vi "StudentScope.vi"() -> ()   [LabVIEW 2015]
uses:
  <vilib>/DAQmx/read.llb/DAQmx Read (Analog 2D DBL NChan NSamp).vi
  <vilib>/DAQmx/create/channels.llb/DAQmx Create Channel (AI-Voltage-Basic).vi
  <vilib>/DAQmx/configure/timing.llb/DAQmx Timing (Sample Clock).vi
  <vilib>/DAQmx/miscellaneous.llb/DAQmx Fill In Error Info.vi
  <resource>/objmgr/daqmx.rc
panel:
  out "Hidden Power Spectrum":T1(graph)=[{"df"=0.0, "df"=2.0, "Power Spectrum (V^2 rms)"=array[5000 elements]}, {"df"=0.0, "df"=2.0, "Power Spectrum (V^2 rms)"=array[5000 elements]}]
  in  "CH B Center":bool
  in  "CH A Center":bool
  out "Hidden Scope":dbl[][](graph)
  out "Acq Rate (Hz)":dbl=20.0 caption="Acq Rate:" format="%#_2g"
  in  "Print":bool
  in  "Tab Control":enum32{"Scope", "Spectrum Analyzer"}(tab)
  out "dV":string="142.75 µs" caption="dV:"
  out "Scope graph":dbl[][](graph)=[[-0.0025862696478761516, 0.003794052366753585, -0.011518720468357783, 0.0025179879638276377, -0.01789904248298752, -0.010242656065431836, -0.016622978080061572, -0.008966591662505888, -0.0025862696478761516, 0.003794052366753585, 0.0025179879638276377, -0.0064144628566539935, -0.0013102052449502043, -0.011518720468357783, -0.003862334050802099, -0.008966591662505888, -0.003862334050802099, -0.0064144628566539935, -0.015346913677135626, 0.0025179879638276377, 0.0012419235609016904, -0.008966591662505888, -0.0064144628566539935, -0.008966591662505888, -0.003862334050802099, -0.003862334050802099, -0.016622978080061572, -0.010242656065431836, -0.0025862696478761516, -0.005138398453728046, -0.011518720468357783, 0.003794052366753585, -0.015346913677135626, -0.015346913677135626, 0.0025179879638276377, -0.0013102052449502043, -0.0064144628566539935, 0.003794052366753585, -0.016622978080061572, 0.0025179879638276377, -0.011518720468357783, -0.008966591662505888, -0.0025862696478761516, -0.008966591662505888, -0.0025862696478761516, -0.01279478487128373, -0.01279478487128373, -0.0013102052449502043, -0.011518720468357783, 0.003794052366753585, -0.0064144628566539935, -0.008966591662505888, -0.015346913677135626, -0.0025862696478761516, -0.003862334050802099, -0.0064144628566539935, -3.4140842024256955e-05, -0.005138398453728046, -0.011518720468357783, -0.005138398453728046, -0.007690527259579941, 0.007622245575531427, -0.007690527259579941, 0.007622245575531427, -0.0064144628566539935, -0.007690527259579941, -0.0025862696478761516, -0.0064144628566539935, -0.0064144628566539935, -0.0064144628566539935, -3.4140842024256955e-05, -0.007690527259579941, -0.01789904248298752, 0.0012419235609016904, -0.0064144628566539935, 0.003794052366753585, -0.011518720468357783, -0.003862334050802099, -0.015346913677135626, 0.003794052366753585, -0.011518720468357783, -0.007690527259579941, 0.005070116769679532, -0.0025862696478761516, -0.0013102052449502043, -0.008966591662505888, -0.003862334050802099, -0.0025862696478761516, -0.015346913677135626, -0.0064144628566539935, 0.0025179879638276377, 0.0012419235609016904, 0.003794052366753585, -0.01279478487128373, -0.016622978080061572, 0.0012419235609016904, -0.005138398453728046, 0.003794052366753585, -0.003862334050802099, -0.005138398453728046, -0.008966591662505888, -0.005138398453728046, 0.003794052366753585, 0.007622245575531427, -0.0064144628566539935, -0.008966591662505888, -0.0013102052449502043, -0.0064144628566539935, 0.014002567590161163, -0.010242656065431836, -0.010242656065431836, -0.008966591662505888, -0.016622978080061572, -0.0025862696478761516, -0.0025862696478761516, 0.005070116769679532, -0.016622978080061572, -0.0013102052449502043, -0.005138398453728046, -0.0013102052449502043, -0.0013102052449502043, 0.003794052366753585, 0.017830760798939006, -0.007690527259579941, -0.020451171288839415, -0.010242656065431836, -0.0013102052449502043, 0.005070116769679532, 0.014002567590161163, 0.007622245575531427, 0.00634618117260548, -0.011518720468357783, -0.0013102052449502043, -0.011518720468357783, -0.0025862696478761516, -0.0064144628566539935, -0.0025862696478761516, -0.0025862696478761516, 0.008898309978457374, 0.00634618117260548, -0.005138398453728046, 0.0025179879638276377, -0.008966591662505888, -0.007690527259579941, 0.005070116769679532, -0.0064144628566539935, 0.005070116769679532, -3.4140842024256955e-05, -0.005138398453728046, 0.0012419235609016904, -0.015346913677135626, 0.003794052366753585, -0.007690527259579941, 0.008898309978457374, 0.0025179879638276377, 0.0025179879638276377, -0.0013102052449502043, -3.4140842024256955e-05, 0.003794052366753585, 0.003794052366753585, -0.003862334050802099, 0.003794052366753585, -0.005138398453728046, -0.0064144628566539935, -0.008966591662505888, -0.0064144628566539935, -0.0013102052449502043, -0.007690527259579941, -3.4140842024256955e-05, -0.003862334050802099, 0.007622245575531427, 0.003794052366753585, 0.003794052366753585, -3.4140842024256955e-05, 0.003794052366753585, 0.003794052366753585, 0.008898309978457374, 0.012726503187235217, 0.0025179879638276377, -0.0025862696478761516, -0.0025862696478761516, -0.003862334050802099, -0.0013102052449502043, -0.0064144628566539935, -0.003862334050802099, 0.0025179879638276377, 0.008898309978457374, 0.005070116769679532, -0.0025862696478761516, 0.00634618117260548, 0.014002567590161163, -0.008966591662505888, 0.008898309978457374, 0.0025179879638276377, 0.014002567590161163, -0.0013102052449502043, 0.003794052366753585, -0.0025862696478761516, 0.01527863199308711, -0.005138398453728046], [-0.00392960120349739, 0.0037154429290138027, 0.0037154429290138027, -0.0013812531593269933, 0.006263790973184202, 0.0037154429290138027, 0.0037154429290138027, 0.006263790973184202, -0.00392960120349739, 0.0037154429290138027, 0.008812139017354599, -0.0013812531593269933, 0.0037154429290138027, 0.0037154429290138027, 0.0011670948848434039, 0.008812139017354599, 0.0037154429290138027, 0.0037154429290138027, 0.008812139017354599, -0.0013812531593269933, 0.0037154429290138027, 0.0037154429290138027, 0.0037154429290138027, 0.006263790973184202, -0.0013812531593269933, 0.0011670948848434039, 0.0037154429290138027, -0.0013812531593269933, 0.006263790973184202, 0.0037154429290138027, 0.0037154429290138027, 0.0011670948848434039, -0.0013812531593269933, 0.006263790973184202, 0.0037154429290138027, 0.0011670948848434039, 0.0037154429290138027, 0.0011670948848434039, 0.006263790973184202, -0.0013812531593269933, 0.0037154429290138027, 0.0011670948848434039, 0.0011670948848434039, 0.011360487061524996, -0.0013812531593269933, 0.0037154429290138027, 0.0037154429290138027, 0.0037154429290138027, 0.008812139017354599, -0.0013812531593269933, 0.011360487061524996, 0.0037154429290138027, 0.0037154429290138027, 0.0037154429290138027, -0.00392960120349739, 0.008812139017354599, -0.0013812531593269933, 0.0037154429290138027, 0.0037154429290138027, 0.0037154429290138027, 0.008812139017354599, 0.0011670948848434039, 0.006263790973184202, -0.00392960120349739, 0.0011670948848434039, 0.0011670948848434039, 0.0037154429290138027, 0.011360487061524996, -0.0013812531593269933, 0.008812139017354599, -0.0013812531593269933, 0.0037154429290138027, 0.0037154429290138027, 0.0037154429290138027, 0.0037154429290138027, -0.0013812531593269933, 0.006263790973184202, -0.0013812531593269933, 0.011360487061524996, 0.0037154429290138027, 0.0037154429290138027, 0.0011670948848434039, 0.0037154429290138027, 0.008812139017354599, -0.0013812531593269933, 0.011360487061524996, -0.006477949247667789, 0.006263790973184202, 0.0037154429290138027, 0.0037154429290138027, 0.006263790973184202, 0.0011670948848434039, 0.0011670948848434039, -0.0013812531593269933, 0.008812139017354599, -0.0013812531593269933, 0.008812139017354599, 0.0011670948848434039, 0.0037154429290138027, 0.0011670948848434039, 0.0037154429290138027, 0.0011670948848434039, 0.0037154429290138027, 0.0037154429290138027, -0.0013812531593269933, 0.008812139017354599, -0.0013812531593269933, 0.008812139017354599, -0.0013812531593269933, 0.0037154429290138027, 0.0037154429290138027, 0.0037154429290138027, 0.0037154429290138027, 0.0037154429290138027, 0.0037154429290138027, 0.0037154429290138027, 0.008812139017354599, -0.0013812531593269933, 0.006263790973184202, -0.0013812531593269933, 0.006263790973184202, 0.0011670948848434039, 0.008812139017354599, 0.0037154429290138027, 0.006263790973184202, 0.0037154429290138027, 0.0037154429290138027, 0.0037154429290138027, 0.0037154429290138027, 0.0037154429290138027, 0.006263790973184202, 0.008812139017354599, -0.0013812531593269933, 0.008812139017354599, -0.0013812531593269933, 0.006263790973184202, -0.0013812531593269933, 0.008812139017354599, 0.0011670948848434039, 0.006263790973184202, 0.0037154429290138027, 0.0037154429290138027, 0.0037154429290138027, 0.0037154429290138027, 0.0037154429290138027, 0.0037154429290138027, 0.006263790973184202, 0.0037154429290138027, 0.0037154429290138027, 0.0037154429290138027, 0.008812139017354599, -0.0013812531593269933, 0.008812139017354599, -0.0013812531593269933, 0.011360487061524996, -0.0013812531593269933, 0.008812139017354599, -0.0013812531593269933, 0.011360487061524996, -0.0013812531593269933, 0.011360487061524996, -0.0013812531593269933, 0.0037154429290138027, 0.0037154429290138027, 0.0037154429290138027, 0.0037154429290138027, 0.0037154429290138027, 0.0037154429290138027, 0.0037154429290138027, 0.0037154429290138027, 0.0037154429290138027, 0.0011670948848434039, 0.0037154429290138027, 0.0037154429290138027, 0.0037154429290138027, 0.0037154429290138027, 0.0037154429290138027, 0.0037154429290138027, 0.0037154429290138027, 0.006263790973184202, -0.0013812531593269933, 0.008812139017354599, -0.00392960120349739, 0.006263790973184202, -0.0013812531593269933, 0.006263790973184202, -0.0013812531593269933, 0.008812139017354599, -0.0013812531593269933, 0.008812139017354599, 0.0011670948848434039, 0.008812139017354599, -0.0013812531593269933, 0.011360487061524996, 0.0011670948848434039, 0.008812139017354599, 0.0011670948848434039, 0.008812139017354599, 0.0011670948848434039, 0.008812139017354599]]
  out "Ch 1 Freq":string="0 kHz" caption="Ch 1 Freq:"
  out "Ch 0 Freq":string="0 Hz" caption="Ch 0 Freq:"
  out "Ch 0 Amp":string="0 V" caption="Ch 0 Amplitude:"
  out "Ch 1 Amp":string="0 V" caption="Ch 1 Amplitude:"
  out "Acq Rate (kHz)":dbl=20.0 caption="Acq Rate:" format="%#_2g"
  out "dT":string="142.75 µs" caption="dt:"
  out "C1 Voltage":string="-4.92 V" caption="C1:"
  out "C2 Voltage":string="-4.91 V" caption="C2:"
  in  "Center Cursor":bool caption="Differential Ch 1"
  out "Ch 0 Amplitude\n(Peak to Peak)":string
  out "Ch 1 Amplitude\n(Peak to Peak)":string
  out "Freq at Cursor":string
  out "Ch 1 Main Freq":string
  out "Ch 0 Main Freq":string
  in  "X Scroll (Hz)":i32(slide)=10000 caption="X Axis Scroll" scale=10.0..50000.0 scale format="%.0p"
  in  "X Axis Zoom":i32(slide)=10000 scale=100.0..10000.0
  out "Power Spectrum":T1(graph)=[{"df"=0.0, "df"=2.0, "Power Spectrum (V^2 rms)"=array[5000 elements]}, {"df"=0.0, "df"=2.0, "Power Spectrum (V^2 rms)"=array[5000 elements]}]
  in  "Input Voltage Range":u16(ring)=2 items=["1 V", "5 V", "10 V", "20 V"]
  in  "Lock Cursors":bool
  out "Rate":dbl=20000.0
  in  "Stop":bool
  in  "Device":dbl=1.0 min=1.0 max=20.0 step=1.0 format="%#_1g"
  in  "Help":bool
  out "Channel A LED":bool=TRUE
  in  "Cursors":bool
  in  "C1 Select":u32(ring) caption="C1" items=["CH 0", "CH 1"]
  in  "Reset":bool
  in  "Log":bool
  in  "CH B Vert Pos":sgl(knob) caption="Position" scale=-10.0..10.0 scale format="%.1f"
  in  "CH A Vert Pos":sgl(knob) caption="Position" scale=-10.0..10.0 scale format="%.1f"
  in  "CH B Zero Pos":bool
  in  "CH A Zero Pos":bool
  in  "CH A Display":bool=TRUE caption="Differental Ch 0"
  in  "Level":dbl caption="V"
  in  "CH 1 Scale":u32(knob)=6 caption="/div" scale=0.0..8.0
  in  "Timebase":i32(knob)=3 caption="/div" scale=0.0..8.0
  in  "CH 0 Scale":u32(knob)=6 caption="/div" scale=0.0..8.0
  in  "Trigger Channel":u16(ring) items=["Channel 0", "Channel 1"]
  in  "Trigger Slope":bool caption="Edge"
  # "Offset"
  # "Offset"
  # "Trigger"
  # "Cursors"
  # "kHz"
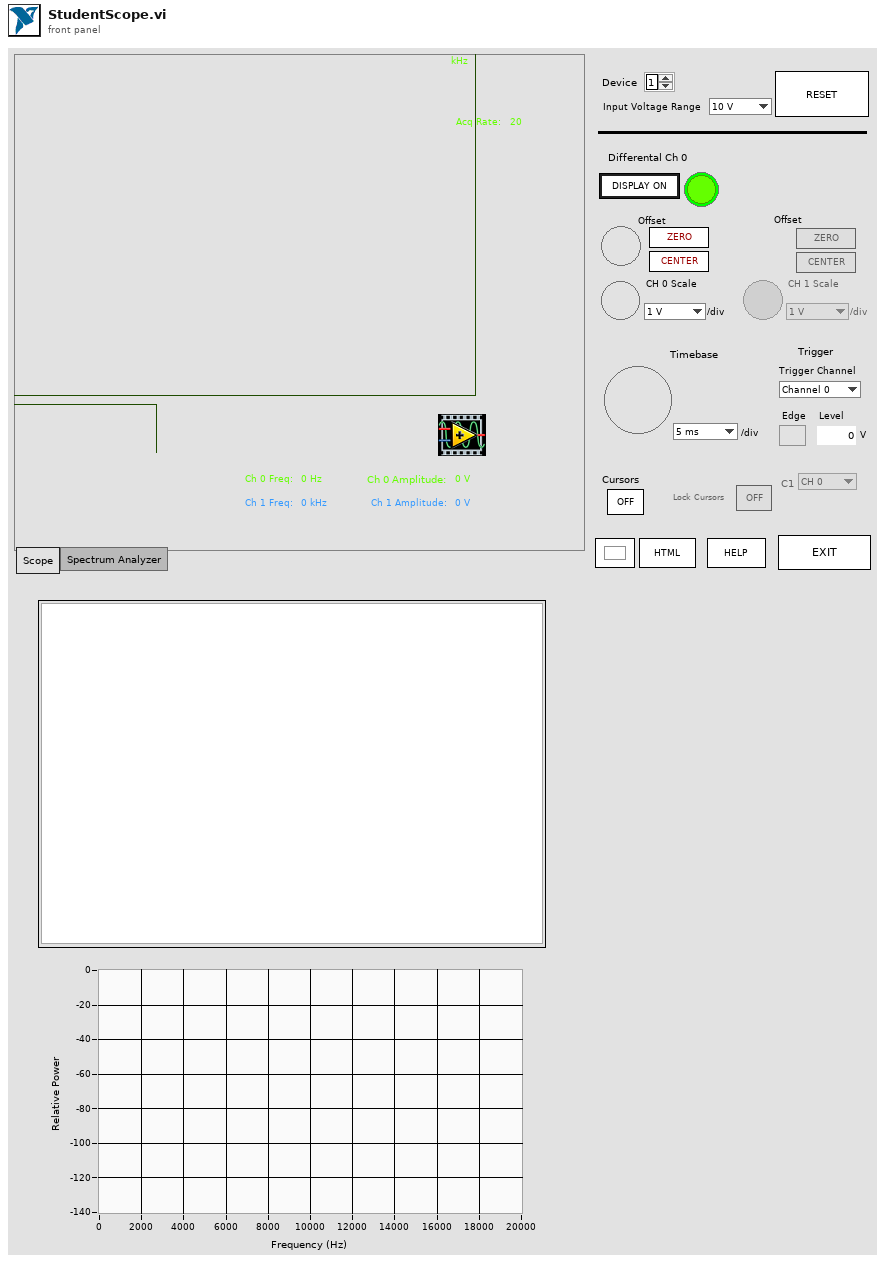
[diagram p1: front panel]
types:
  T1 = cluster{"df":dbl, "df":dbl, "Power Spectrum (V^2 rms)":dbl[]}[]
  T2 = cluster{"Minimum":dbl, "Maximum":dbl, "Increment":dbl, "Minor Incr":dbl, "Start":dbl}
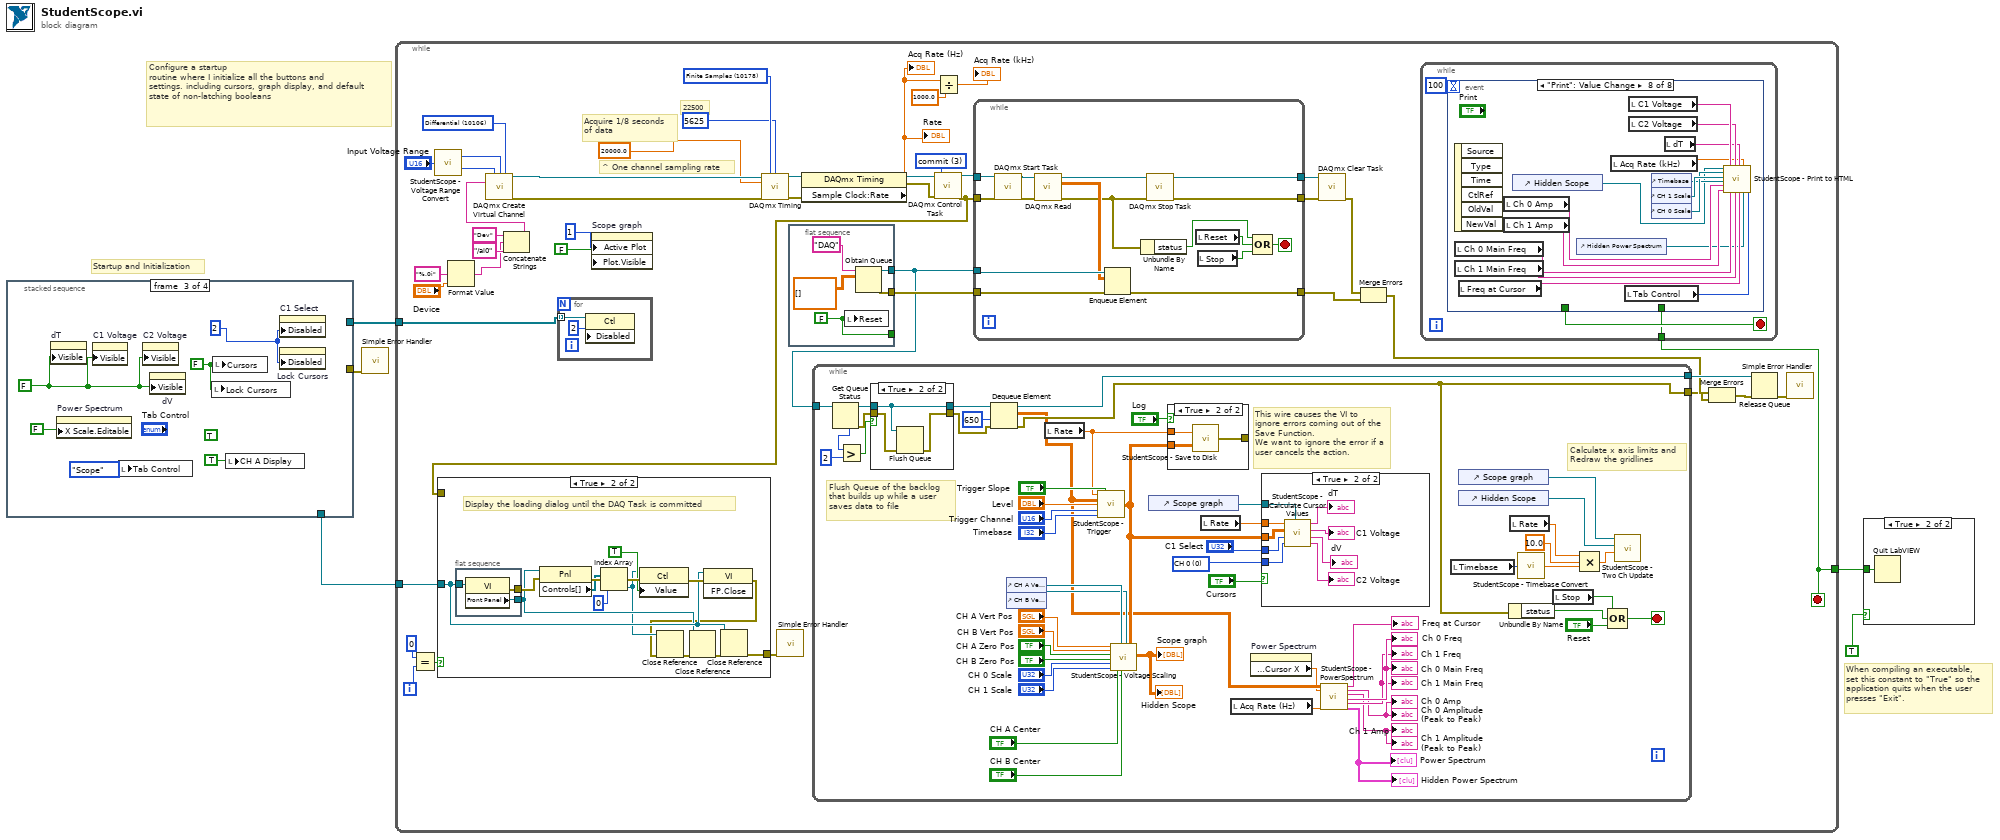
[diagram p0: block diagram]
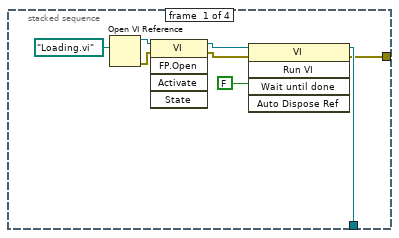
[diagram p3: hidden frame]
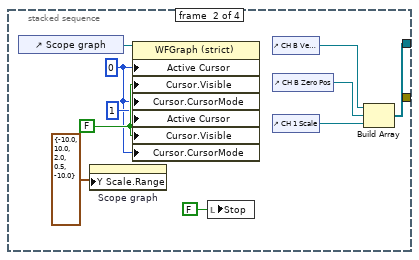
[diagram p4: hidden frame]
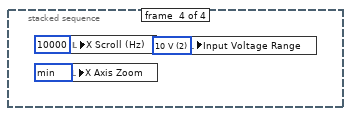
[diagram p5: hidden frame]
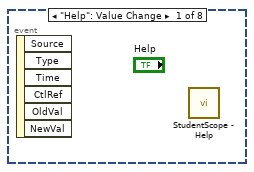
[diagram p7: hidden frame]
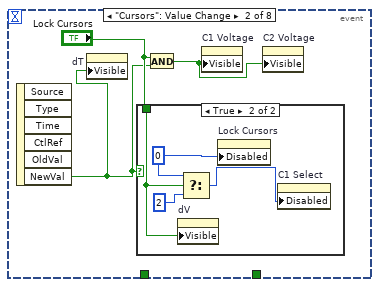
[diagram p8: hidden frame]
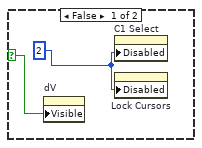
[diagram p9: hidden frame]
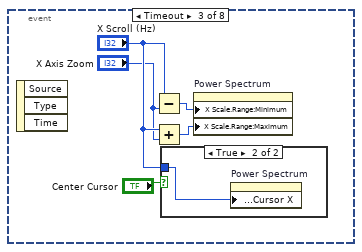
[diagram p10: hidden frame]
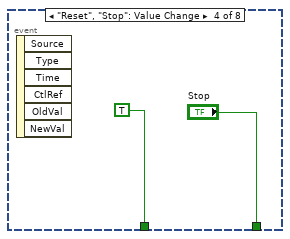
[diagram p12: hidden frame]
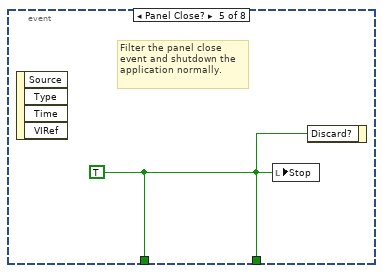
[diagram p13: hidden frame]
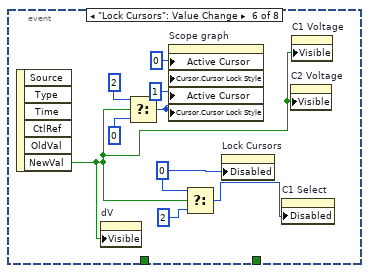
[diagram p14: hidden frame]
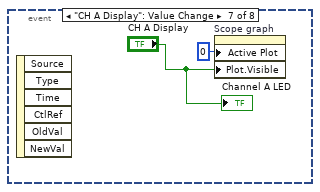
[diagram p15: hidden frame]
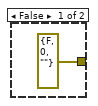
[diagram p17: hidden frame]
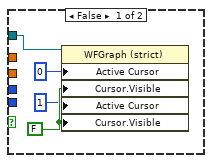
[diagram p18: hidden frame]
diagram:
  # "When compiling an executable, set this constant to \"True\" so the application quits when the user presses \"Exit\"."
  # "Startup and Initialization"
  # "Configure a startup\nroutine where I initialize all the buttons and\nsettings. including cursors, graph display, and default\nstate of non-latching booleans"
  n1 = stacked-sequence {
    tunnel: [_ w15 _ _] -> w5
    tunnel: [w7 _ _ _] -> w3
    tunnel: [w6 _ _ _] -> w4
    frame #0 {
      n2 = Open VI Reference(vi path=path "Loading.vi") -> (vi reference=w11:refnum<vi>, error out=w10:errorcluster)  [unwired: 5 in]
      n3 = invoke class="VI" method="FP.Open"(reference=w11, error in=w10) -> (reference out=w9:refnum<vi>, error out=w8:errorcluster)  [unwired: 3 in, 3 out]
      n4 = invoke class="VI" method="Run VI"(reference=w9, error in=w8, "Wait until done"=FALSE) -> (reference out=w7:refnum<vi>, error out=w6:errorcluster)  [unwired: 2 in, 3 out]
    }
    frame #1 {
      w17 = FALSE ("Cursor.Visible")
      w14 = u32 0 ("Active Cursor")
      n5 = control-ref of="Scope graph"() -> (w18:refnum<vi>)
      n6 = property on="Scope graph" class="WFGraph (strict)"("Y Scale.Range"=T2 {"Minimum"=-10.0, "Maximum"=10.0, "Increment"=2.0, "Minor Incr"=0.5, "Start"=-10.0}) -> ()  [unwired: 2 in, 2 out]
      n7 = property class="WFGraph (strict)"(reference=w18, "Active Cursor"=w14, "Cursor.Visible"=w17, "Cursor.CursorMode"=w14, "Active Cursor"=u32 1, "Cursor.Visible"=w17, "Cursor.CursorMode"=w14) -> ()  [unwired: 1 in, 2 out]
      n8 = local write "Stop"(FALSE ("stop")) -> ()
      n9 = control-ref of="CH B Vert Pos"() -> (w22:refnum<vi>)
      n10 = control-ref of="CH B Zero Pos"() -> (w21:refnum<vi>)
      n11 = control-ref of="CH 1 Scale"() -> (w20:refnum<vi>)
      n12 = Build Array(w22, w21, w20) -> (w15:refnum<vi>[])
    }
    frame #2 {
      (unwired) TRUE ("CH B Display")
      w28 = FALSE ("Cursors")
      w24 = FALSE ("Visible")
      w29 = u8 2 ("Disabled")
      n13 = property on="dT" class="Str"("Visible"=w24) -> ()  [unwired: 2 in, 2 out]
      n14 = property on="Power Spectrum" class="WFGraph (strict)"("X Scale.Editable"=FALSE) -> ()  [unwired: 2 in, 2 out]
      n15 = property on="C1 Voltage" class="Str"("Visible"=w24) -> ()  [unwired: 2 in, 2 out]
      n16 = local write "Tab Control"(enum32{"Scope", "Spectrum Analyzer"}."Scope" ("Tab Control")) -> ()
      n17 = property on="C2 Voltage" class="Str"("Visible"=w24) -> ()  [unwired: 2 in, 2 out]
      n18 = property on="dV" class="Str"("Visible"=w24) -> ()  [unwired: 2 in, 2 out]
      n19 = local write "Lock Cursors"(w28) -> ()
      n20 = local write "Cursors"(w28) -> ()
      n21 = local write "CH A Display"(TRUE ("CH B Display")) -> ()
      n22 = property on="C1 Select" class="Ring (strict)"("Disabled"=w29) -> ()  [unwired: 2 in, 2 out]
      n23 = property on="Lock Cursors" class="Bool (strict)"("Disabled"=w29) -> ()  [unwired: 2 in, 2 out]
    }
    frame #3 {
      w30 = u16 2 items=["1 V", "5 V", "10 V", "20 V"] ("Input Voltage Range")
      w31 = 10000 items=["min"=10000, ""=1000, "max"=100] ("X Axis Zoom")
      n24 = local write "X Axis Zoom"(w31) -> ()
      n25 = local write "X Scroll (Hz)"(10000 ("X Scroll (Hz)")) -> ()
      n26 = local write "Input Voltage Range"(w30) -> ()
    }
  }
  n27 = call <vilib>:"Simple Error Handler.vi"("error in (no error)"=w4) -> ()  [unwired: 4 in, 5 out]
  n28 = while {
    tunnel: w5 -> [w45]
    tunnel: w3 -> [w44]
    tunnel: [w42] -> w2
    i -> [w48]
    stop <- w42 stop-if-true
    w65 = 10178 items=["Finite Samples"=10178, "Continuous Samples"=10123, "Hardware Timed Single Point"=12522] ("sample mode")
    w72 = 3 items=["verify"=2, "reserve"=4, "commit"=3, "unreserve"=5, "abort"=6] ("action")
    w76 = 10106 items=["default"=-1, "RSE"=10083, "NRSE"=10078, "Differential"=10106, "Pseudodifferential"=12529] ("input terminal configuration")
    # "22500"
    # "^ One channel sampling rate"
    # "Acquire 1/8 seconds\nof data"
    n29 = Equal?(x=0, y=w48) -> (x = y?=w46:bool)
    n30 = call "StudentScope - Voltage Range Convert.vi"("Input Voltage Range"="Input Voltage Range") -> ("V min"=w51:i32, "V max"=w50:i32)
    n31 = Format Value(format string="%.0i", value (0)="Device") -> (output string=w59:string)  [unwired: 1 in]
    n32 = Concatenate Strings("Dev" ("string"), w59, "/ai0" ("string")) -> (w67:string)
    n33 = call-poly <vilib>:"DAQmx Create Virtual Channel.vi"("maximum value"=w50, "minimum value"=w51, "input terminal configuration"=w76, "physical channels"=w67) -> ("task out"=w77:refnum<k21>, "error out"=w64:errorcluster)  [unwired: 10 in]
    n34 = for {
      tunnel: w45 -> [w78] mode=indexing
      n35 = property class="Ctl"(reference=w78, "Disabled"=u8 2) -> ()  [unwired: 1 in, 2 out]
    }
    n36 = property on="Scope graph" class="WFGraph (strict)"("Active Plot"=u32 1, "Plot.Visible"=FALSE) -> ()  [unwired: 2 in, 2 out]
    n37 = call-poly <vilib>:"DAQmx Timing.vi"("task/channels in"=w77, "sample mode"=w65, "samples per channel"=5625, "rate"=20000.0 ("minimum value"), "error in"=w64) -> ("task out"=w66:refnum<k21>, "error out"=w55:errorcluster)  [unwired: 9 in]
    n38 = flat-sequence {
      tunnel: [w147] -> _
      tunnel: [w144] -> w56
      tunnel: [w143] -> w58
      frame #0 {
        w147 = FALSE ("stop")
        n39 = local write "Reset"(w147) -> ()
        n40 = Obtain Queue(name (unnamed)="DAQ", element data type=dbl[][] [] ("data")) -> (queue out=w144:refnum<queue>, error out=w143:errorcluster)  [unwired: 3 in, 1 out]
      }
    }
    n41 = property class="DAQmx Timing"(reference=w66, error in=w55) -> (reference out=w53:refnum<k21>, error out=w54:errorcluster, "Sample Clock:Rate"=w41:dbl)
    "Rate" <- w41
    "Acq Rate (Hz)" <- w41
    n42 = while {
      tunnel: w56 -> [w165]
      tunnel: [w180] -> w62
      tunnel: [w178] -> w37
      stop <- w182 stop-if-true
      w183 = u32 0 items=["CH 0", "CH 1"] ("C2 Select")
      # "This wire causes the VI to ignore errors coming out of the Save Function.\nWe want to ignore the error if a user cancels the action."
      # "Flush Queue of the backlog\nthat builds up while a user\nsaves data to file"
      # "Calculate x axis limits and\nRedraw the gridlines"
      n43 = Get Queue Status(queue=w165) -> (queue out=w168:refnum<queue>, error out=w163:errorcluster, # elements in queue=w164:i32)  [unwired: 2 in, 5 out]
      n44 = Greater?(x=w164, y=2) -> (0:w166:bool)
      n45 = case shown="True" w166 {
        tunnel: [w203 w206] -> w169
        tunnel: w168 -> [w203 w206]
        tunnel: w163 -> [w202 w205]
        tunnel: [w202 w204] -> w162
        frame False {
        }
        frame True {
          n46 = Flush Queue(queue=w206, error in (no error)=w205) -> (error out=w204:errorcluster)  [unwired: 2 out]
        }
      }
      n47 = Dequeue Element(queue=w169, timeout in ms (-1)=650, error in (no error)=w162) -> (queue out=w180:refnum<queue>, element=w159:dbl[][], error out=w178:errorcluster)  [unwired: 1 out]
      n48 = control-ref of="CH A Vert Pos"() -> (w191:refnum<vi>)
      n49 = control-ref of="CH B Vert Pos"() -> (w190:refnum<vi>)
      n50 = local read "Rate"() -> (w185:dbl)
      n51 = call "StudentScope - Trigger.vi"("Rate"=w185, "Trigger Slope"="Trigger Slope", "data"=w159, "Level"="Level", "Trigger Channel"="Trigger Channel", "Sec/Div"="Timebase") -> ("Array"=w160:dbl[][])  [unwired: 9 in]
      n52 = call "StudentScope - Voltage Scaling.vi"("CH A Vert Pos"="CH A Vert Pos", "CH B Vert Pos"="CH B Vert Pos", "CH A Zero Pos"="CH A Zero Pos", "CH B Zero Pos"="CH B Zero Pos", "CH A Scale"="CH 0 Scale", "CH B Scale"="CH 1 Scale", "CH A Center"="CH A Center", "Knob A Refnum"=w191, "CH B Center"="CH B Center", "Knob B Refnum"=w190, "Raw Y Values"=w160) -> ("Scaled Y Values"=→"Scope graph" →"Hidden Scope":dbl[][])  [unwired: 8 in]
      n53 = control-ref of="Scope graph"() -> (w188:refnum<vi>)
      n54 = case shown="True" "Log" {
        tunnel: w160 -> [_ w209]
        tunnel: w185 -> [_ w210]
        tunnel: [errorcluster {"status"=FALSE, "code"=0, "source"=""} ("error out") w208] -> _
        frame False {
        }
        frame True {
          n55 = call "StudentScope - Save to Disk.vi"("Y Values"=w209, "Rate"=w210) -> ("error out"=w208:errorcluster)  [unwired: 1 in]
        }
      }
      n56 = local read "Rate"() -> (w187:dbl)
      n57 = local read "Acq Rate (Hz)"() -> (w161:dbl)
      n58 = property on="Power Spectrum" class="WFGraph (strict)"() -> ("Cursor.Cursor Position:Cursor X"=w155:dbl)  [unwired: 2 in, 2 out]
      n59 = case shown="True" "Cursors" {
        tunnel: w160 -> [_ w222]
        tunnel: w188 -> [w211 w216]
        tunnel: w187 -> [_ w223]
        tunnel: "C1 Select" -> [_ w221]
        tunnel: w183 -> [_ w220]
        frame False {
          w213 = FALSE ("Cursor.Visible")
          n60 = property class="WFGraph (strict)"(reference=w211, "Active Cursor"=u32 0, "Cursor.Visible"=w213, "Active Cursor"=u32 1, "Cursor.Visible"=w213) -> ()  [unwired: 1 in, 2 out]
        }
        frame True {
          n61 = call "StudentScope - Calculate Cursor Values.vi"("Scope graph"=w216, "C2 Select"=w220, "C1 Select"=w221, "Array"=w222, "Rate"=w223) -> ("C2 Voltage"=→"C2 Voltage":string, "dV"=→"dV":string, "C1 Voltage"=→"C1 Voltage":string, "dT"=→"dT":string)  [unwired: 1 in]
        }
      }
      n62 = call "StudentScope - PowerSpectrum.vi"("data"=w159, "Cursor Position"=w155, "Acq Rate (Hz)"=w161) -> ("Cursor Freq"=→"Freq at Cursor":string, "Ch0 Amp"=→"Ch 0 Amp" →"Ch 0 Amplitude\n(Peak to Peak)":string, "Ch1 Amp"=→"Ch 1 Amp" →"Ch 1 Amplitude\n(Peak to Peak)":string, "Ch0 Freq"=→"Ch 0 Main Freq" →"Ch 0 Freq":string, "Ch1 Freq"=→"Ch 1 Main Freq" →"Ch 1 Freq":string, "Normalized Power Spectrum"=→"Power Spectrum" →"Hidden Power Spectrum":cluster{"df":dbl, "df":dbl, "Y":dbl[]}[])  [unwired: 11 in]
      n63 = local read "Timebase"() -> (w175:i32)
      n64 = control-ref of="Scope graph"() -> (w172:refnum<vi>)
      n65 = control-ref of="Hidden Scope"() -> (w151:refnum<vi>)
      n66 = Unbundle By Name(w178) -> ("status"=w177:bool)
      n67 = local read "Rate"() -> (w171:dbl)
      n68 = call "StudentScope - Timebase Convert.vi"("Sec/Div"=w175) -> ("Sec/Div"=w174:dbl)
      n69 = local read "Stop"() -> (w176:bool)
      n70 = Compound Arithmetic op=MULTIPLY(w171, 10.0 ("Rate"), w174) -> (w173:dbl)
      n71 = Compound Arithmetic op=OR(w176, w177, "Reset") -> (w182:bool)
      n72 = call "StudentScope - Two Ch Update.vi"("Samples/Graph"=w173, "scope graph ref 2"=w151, "scope graph ref"=w172) -> ()  [unwired: 9 in]
    }
    n73 = call <vilib>:"DAQmx Control Task.vi"("task/channels in"=w53, "action"=w72, "error in"=w54) -> ("task out"=w73:refnum<k21>, "error out"=w49:errorcluster)  [unwired: 11 in]
    n74 = case shown="True" w46 {
      tunnel: w49 -> [_ _]
      tunnel: w44 -> [_ w86]
      tunnel: [_ w85] -> w43
      frame False {
      }
      frame True {
        # "Display the loading dialog until the DAQ Task is committed"
        n75 = flat-sequence {
          tunnel: [w95] -> w87
          tunnel: [w94] -> w84
          tunnel: w86 -> [w93]
          frame #0 {
            n76 = property class="VI"(reference=w93) -> (error out=w95:errorcluster, "Front Panel"=w94:refnum<vi>)  [unwired: 1 in, 1 out]
          }
        }
        n77 = property class="Pnl"(reference=w84, error in=w87) -> (error out=w91:errorcluster, "Controls[]"=w90:refnum<vi>[])  [unwired: 1 out]
        n78 = Index Array(array=w90, index=0) -> (element=w81:refnum<vi>)
        n79 = property class="Ctl"(reference=w81, error in=w91, "Value"=TRUE) -> (error out=w92:errorcluster)  [unwired: 1 out]
        n80 = invoke class="VI" method="FP.Close"(reference=w86, error in=w92) -> (error out=w80:errorcluster)  [unwired: 1 in, 2 out]
        n81 = Close Reference(reference=w81, error in (no error)=w80) -> (error out=w82:errorcluster)
        n82 = Close Reference(reference=w84, error in (no error)=w82) -> (error out=w83:errorcluster)
        n83 = Close Reference(reference=w86, error in (no error)=w83) -> (error out=w85:errorcluster)
      }
    }
    n84 = call <vilib>:"Simple Error Handler.vi"("error in (no error)"=w43) -> ()  [unwired: 4 in, 5 out]
    n85 = Divide(x=w41, y=1000.0) -> (x/y=→"Acq Rate (kHz)":dbl)
    n86 = while {
      tunnel: w73 -> [w239]
      tunnel: w49 -> [w225]
      tunnel: [w228] -> w74
      tunnel: w56 -> [w238]
      tunnel: w58 -> [w237]
      tunnel: [w236] -> w39
      tunnel: [w230] -> w75
      stop <- w235 stop-if-true
      n87 = call <vilib>:"DAQmx Start Task.vi"("task/channels in"=w239, "error in"=w225) -> ("task out"=w227:refnum<k21>, "error out"=w226:errorcluster)  [unwired: 12 in]
      n88 = call-poly <vilib>:"DAQmx Read.vi"("task/channels in"=w227, "error in"=w226) -> ("task out"=w231:refnum<k21>, "data"=w234:dbl[][], "error out"=w229:errorcluster)  [unwired: 11 in]
      n89 = Enqueue Element(queue=w238, element=w234, error in (no error)=w237) -> (error out=w236:errorcluster)  [unwired: 1 in, 2 out]
      n90 = Unbundle By Name(w229) -> ("status"=w233:bool)
      n91 = call <vilib>:"DAQmx Stop Task.vi"("task/channels in"=w231, "error in"=w229) -> ("task out"=w230:refnum<k21>, "error out"=w228:errorcluster)  [unwired: 12 in]
      n92 = local read "Reset"() -> (w232:bool)
      n93 = local read "Stop"() -> (w224:bool)
      n94 = Compound Arithmetic op=OR(w233, w232, w224) -> (w235:bool)
    }
    n95 = call <vilib>:"DAQmx Clear Task.vi"("task in"=w75, "error in"=w74) -> ("error out"=w40:errorcluster)  [unwired: 13 in]
    n96 = Merge Errors(w40, w39) -> (w38:errorcluster)
    n97 = while {
      tunnel: [w97] -> w42
      stop <- w98 stop-if-true
      n98 = event shown="[7] \"Print\": Value Change" {
        selector: _ -> [_ _ _ _ _ _ _ _]
        dyn-events: _ -> [_ _ _ _ _ _ _ _]
        timeout: u32 100 ("milliseconds to wait") -> [_ _ _ _ _ _ _ _]
        tunnel: [_ _ _ TRUE ("NewVal") w116 _ _ _] -> w98
        tunnel: [_ _ _ "Stop" w116 _ _ _] -> w97
        event "Help": Value Change {
          n99 = event-data() -> ()  [unwired: 1 in, 6 out]
          n100 = call "StudentScope - Help.vi"() -> ()  [unwired: 1 in]
        }
        event "Cursors": Value Change {
          n101 = event-data() -> ("NewVal"=w99:bool)  [unwired: 1 in, 5 out]
          n102 = property on="dT" class="Str"("Visible"=w99) -> ()  [unwired: 2 in, 2 out]
          n103 = case shown="True" w99 {
            selector: w99 -> [w102 _]
            tunnel: "Lock Cursors" -> [_ w104]
            frame False {
              w103 = u8 2 ("Disabled")
              n104 = property on="dV" class="Str"("Visible"=w102) -> ()  [unwired: 2 in, 2 out]
              n105 = property on="C1 Select" class="Ring (strict)"("Disabled"=w103) -> ()  [unwired: 2 in, 2 out]
              n106 = property on="Lock Cursors" class="Bool (strict)"("Disabled"=w103) -> ()  [unwired: 2 in, 2 out]
            }
            frame True {
              w105 = u8 0 ("Disabled")
              n107 = property on="dV" class="Str"("Visible"=w104) -> ()  [unwired: 2 in, 2 out]
              n108 = Select(t=w105, s=w104, f=u8 2) -> (s? t:f=w106:u8)
              n109 = property on="Lock Cursors" class="Bool (strict)"("Disabled"=w105) -> ()  [unwired: 2 in, 2 out]
              n110 = property on="C1 Select" class="Ring (strict)"("Disabled"=w106) -> ()  [unwired: 2 in, 2 out]
            }
          }
          n111 = And(x="Lock Cursors", y=w99) -> (x .and. y?=w101:bool)
          n112 = property on="C1 Voltage" class="Str"("Visible"=w101) -> ()  [unwired: 2 in, 2 out]
          n113 = property on="C2 Voltage" class="Str"("Visible"=w101) -> ()  [unwired: 2 in, 2 out]
        }
        event Timeout {
          n114 = event-data() -> ()  [unwired: 1 in, 3 out]
          n115 = Subtract(x="X Scroll (Hz)", y="X Axis Zoom") -> (x-y=w110:i32)
          n116 = Add(x="X Scroll (Hz)", y="X Axis Zoom") -> (x+y=w109:i32)
          n117 = case shown="True" "Center Cursor" {
            tunnel: "X Scroll (Hz)" -> [_ w113]
            frame False {
            }
            frame True {
              n118 = property on="Power Spectrum" class="WFGraph (strict)"("Cursor.Cursor Position:Cursor X"=w113) -> ()  [unwired: 2 in, 2 out]
            }
          }
          n119 = property on="Power Spectrum" class="WFGraph (strict)"("X Scale.Range:Minimum"=w110, "X Scale.Range:Maximum"=w109) -> ()  [unwired: 2 in, 2 out]
        }
        event "Reset", "Stop": Value Change {
          n120 = event-data() -> ()  [unwired: 1 in, 6 out]
        }
        event Panel Close? {
          w116 = TRUE
          # "Filter the panel close event and shutdown the application normally."
          n121 = event-data() -> ()  [unwired: 1 in, 4 out]
          n122 = local write "Stop"(w116) -> ()
          n123 = event-data("Discard?"=w116) -> ()  [unwired: 1 in, 1 out]
        }
        event "Lock Cursors": Value Change {
          w118 = u8 0 ("Disabled")
          n124 = event-data() -> ("NewVal"=w117:bool)  [unwired: 1 in, 5 out]
          n125 = property on="dV" class="Str"("Visible"=w117) -> ()  [unwired: 2 in, 2 out]
          n126 = Select(t=u32 2 ("Active Cursor"), s=w117, f=u32 0 ("Active Cursor")) -> (s? t:f=w121:u32)
          n127 = property on="Scope graph" class="WFGraph (strict)"("Active Cursor"=u32 0, "Cursor.Cursor Lock Style"=w121, "Active Cursor"=u32 1, "Cursor.Cursor Lock Style"=w121) -> ()  [unwired: 2 in, 2 out]
          n128 = Select(t=w118, s=w117, f=u8 2) -> (s? t:f=w119:u8)
          n129 = property on="Lock Cursors" class="Bool (strict)"("Disabled"=w118) -> ()  [unwired: 2 in, 2 out]
          n130 = property on="C1 Select" class="Ring (strict)"("Disabled"=w119) -> ()  [unwired: 2 in, 2 out]
          n131 = property on="C2 Voltage" class="Str"("Visible"=w117) -> ()  [unwired: 2 in, 2 out]
          n132 = property on="C1 Voltage" class="Str"("Visible"=w117) -> ()  [unwired: 2 in, 2 out]
        }
        event "CH A Display": Value Change {
          n133 = event-data() -> ()  [unwired: 1 in, 6 out]
          n134 = property on="Scope graph" class="WFGraph (strict)"("Active Plot"=u32 0, "Plot.Visible"="CH A Display") -> ()  [unwired: 2 in, 2 out]
          "Channel A LED" <- "CH A Display"
        }
        event "Print": Value Change {
          n135 = event-data() -> ()  [unwired: 1 in, 6 out]
          n136 = local read "Ch 0 Main Freq"() -> (w134:string)
          n137 = local read "Ch 1 Main Freq"() -> (w133:string)
          n138 = local read "Freq at Cursor"() -> (w135:string)
          n139 = local read "Ch 0 Amp"() -> (w132:string)
          n140 = local read "Ch 1 Amp"() -> (w131:string)
          n141 = control-ref of="Hidden Scope"() -> (w130:refnum<vi>)
          n142 = control-ref of="Hidden Power Spectrum"() -> (w128:refnum<vi>)
          n143 = local read "Acq Rate (kHz)"() -> (w137:dbl)
          n144 = local read "Tab Control"() -> (w129:enum32{"Scope", "Spectrum Analyzer"})
          n145 = local read "C1 Voltage"() -> (w140:string)
          n146 = local read "C2 Voltage"() -> (w139:string)
          n147 = control-ref of="Timebase"() -> (w136:refnum<vi>)
          n148 = control-ref of="CH 1 Scale"() -> (w142:refnum<vi>)
          n149 = control-ref of="CH 0 Scale"() -> (w141:refnum<vi>)
          n150 = local read "dT"() -> (w138:string)
          n151 = call "StudentScope - Print to HTML.vi"("Scope graph"=w130, "CH 0 Scale"=w141, "CH 1 Scale"=w142, "Timebase"=w136, "Ch0 Amp"=w132, "Ch1 Amp"=w131, "C1"=w140, "Ch0 Freq"=w134, "C2"=w139, "Ch1 Freq"=w133, "dT"=w138, "Freq Cursor"=w135, "Acq Rate (kHz)"=w137, "Power Spectrum"=w128, "Tab Control 2"=w129) -> ()  [unwired: 5 in]
        }
      }
    }
    n152 = Merge Errors(w38, w37) -> (w36:errorcluster)
    n153 = Release Queue(queue=w62, error in (no error)=w36) -> (error out=w35:errorcluster)  [unwired: 1 in, 2 out]
    n154 = call <vilib>:"Simple Error Handler.vi"("error in (no error)"=w35) -> ()  [unwired: 4 in, 5 out]
  }
  n155 = case shown="True" TRUE {
    tunnel: w2 -> [_ w240]
    frame False {
    }
    frame True {
      n156 = Quit LabVIEW(quit? (T)=w240) -> ()
    }
  }
